vi "Check Channel.vi"(7 "Peripheral":T7, 8 "Error In":errorcluster, 10 "Channels":u8[](array[numeric]), 11 "LINX Resource":T1) -> (0 "Error Out":errorcluster, 2 "Channels":u8[](array[numeric]), 3 "LINX Resource":T1)   [LabVIEW 2014, in "LMH-LINX.lvlib"]
doc: "Generate an error if the specified peripheral channel does not exist on the LINX device."
uses:
  <vilib>/MakerHub/LINX/LMH-LINX.lvlib
  <vilib>/MakerHub/LINX/Private/Type Defs/Peripheral.ctl
  <vilib>/MakerHub/LINX/Private/Type Defs/LINX Ref.ctl
  <vilib>/MakerHub/LINX/Private/Type Defs/Platform.ctl
  <vilib>/MakerHub/LINX/Private/Type Defs/Interface.ctl
  <vilib>/MakerHub/LINX/Private/Device/Type Defs/LINX Device Config.ctl
  <vilib>/MakerHub/LINX/Private/Device/Type Defs/TCP Config.ctl
  <vilib>/MakerHub/LINX/Private/Device/Type Defs/Channels.ctl
  <vilib>/MakerHub/LINX/Private/Type Defs/Error Type.ctl
  <vilib>/MakerHub/LINX/Private/Device/Device.lvlib
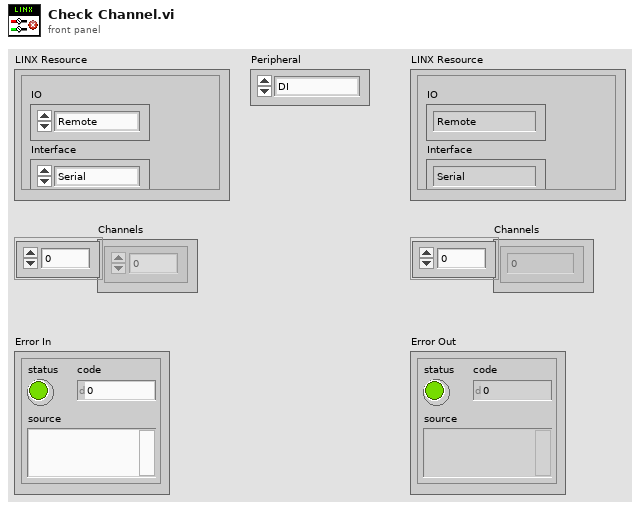
[diagram p1: front panel]
types:
  T1 = typedef "LMH-LINX.lvlib/LINX Ref.ctl" = cluster{"IO":T2, "Interface":T3, "LINX Device Config":T4}
  T2 = typedef "LMH-LINX.lvlib/Platform.ctl" = enum16{"Remote", "Local"}
  T3 = typedef "LMH-LINX.lvlib/Interface.ctl" = enum16{"Serial", "TCP"}
  T4 = typedef "LMH-LINX.lvlib/Device.lvlib/LINX Device Config.ctl" = cluster{"Interface":T3, "COM Port":refnum<visa-resource-name>, "TCP Configuration":T5, "Device Family":u8, "Device ID":u8, "Device Name":string, "TCP Ref":refnum<k5>, "Channels":T6}
  T5 = typedef "LMH-LINX.lvlib/Device.lvlib/TCP Config.ctl" = cluster{"IP Address":string, "Port":u16}
  T6 = typedef "LMH-LINX.lvlib/Channels.ctl" = cluster{"DI":u8[], "DO":u8[], "AI":u8[], "AO":u8[], "PWM":u8[], "QE":u8[], "UART":u8[], "I2C 2":u8[], "SPI":u8[], "CAN":u8[], "Servo":u8[], "AI Ref (V)":dbl, "AI Resolution (Bits)":u8, "AO Ref (V)":dbl, "AO Resolution (Bits)":u8}
  T7 = typedef "LMH-LINX.lvlib/Peripheral.ctl" = enum8{"DI", "DO", "AI", "AO", "PWM", "QE", "UART", "I2C", "SPI", "CAN", "Servo"}
  T8 = typedef "LMH-LINX.lvlib/Error Type.ctl" = enum16{"Unknown", "Timeout", "Corrupt Return Packet", "Unable To Connect", "Command Not Supported", "Channel DNE", "Invalid COM Config", "Firmware Version Mismatch", "myRIO Support", "CMD Specific Error", "Local IO Not Supported"}
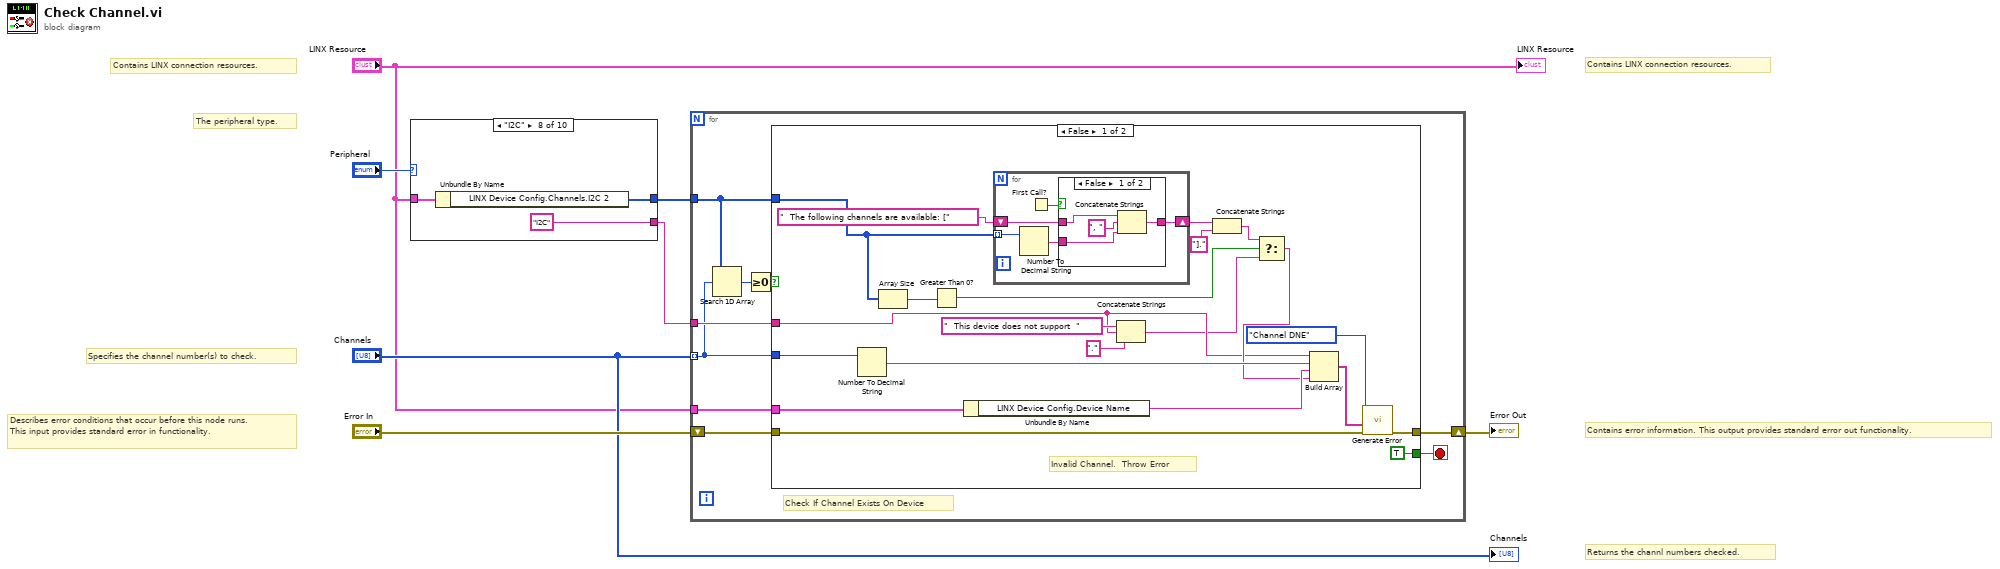
[diagram p0: block diagram]
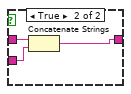
[diagram p2: hidden frame]
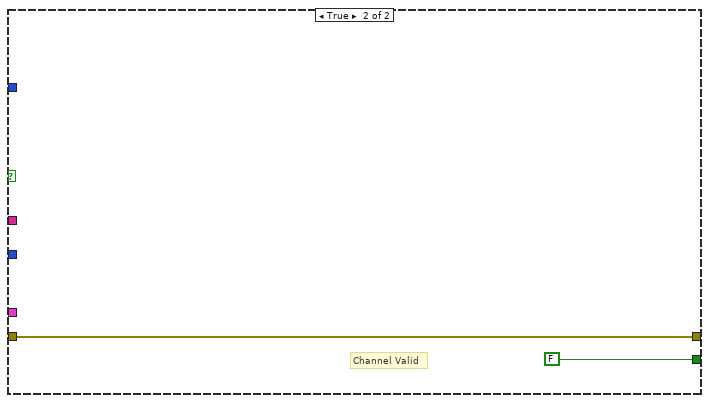
[diagram p3: hidden frame]
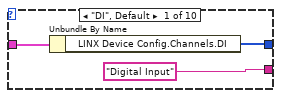
[diagram p4: hidden frame]
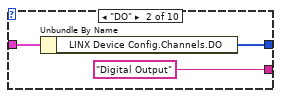
[diagram p5: hidden frame]
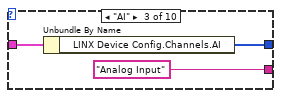
[diagram p6: hidden frame]
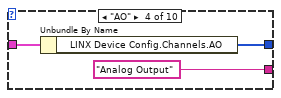
[diagram p7: hidden frame]
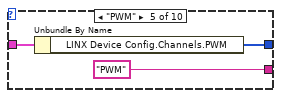
[diagram p8: hidden frame]
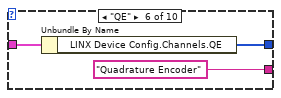
[diagram p9: hidden frame]
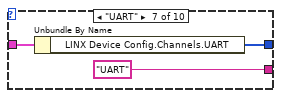
[diagram p10: hidden frame]
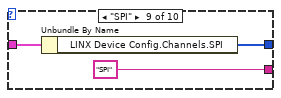
[diagram p11: hidden frame]
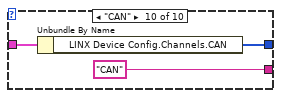
[diagram p12: hidden frame]
diagram:
  # "Returns the channl numbers checked."
  # "Contains LINX connection resources."
  # "Specifies the channel number(s) to check."
  # "The peripheral type."
  # "Contains error information. This output provides standard error out functionality."
  # "Contains LINX connection resources."
  # "Describes error conditions that occur before this node runs. This input provides standard error in functionality."
  n1 = case shown="\"I2C\"" "Peripheral" {
    tunnel: "LINX Resource" -> [w10 w13 w16 w19 w22 w25 w28 w31 w34 w37]
    tunnel: [w9 w12 w15 w18 w21 w24 w27 w30 w33 w36] -> w6
    tunnel: ["Digital Input" "Digital Output" "Analog Input" "Analog Output" "PWM" "Quadrature Encoder" "UART" "I2C" "SPI" "CAN"] -> w4
    frame "DI", Default {
      n2 = Unbundle By Name(w10) -> ("LINX Device Config.Channels.DI"=w9:u8[])
    }
    frame "DO" {
      n3 = Unbundle By Name(w13) -> ("LINX Device Config.Channels.DO"=w12:u8[])
    }
    frame "AI" {
      n4 = Unbundle By Name(w16) -> ("LINX Device Config.Channels.AI"=w15:u8[])
    }
    frame "AO" {
      n5 = Unbundle By Name(w19) -> ("LINX Device Config.Channels.AO"=w18:u8[])
    }
    frame "PWM" {
      n6 = Unbundle By Name(w22) -> ("LINX Device Config.Channels.PWM"=w21:u8[])
    }
    frame "QE" {
      n7 = Unbundle By Name(w25) -> ("LINX Device Config.Channels.QE"=w24:u8[])
    }
    frame "UART" {
      n8 = Unbundle By Name(w28) -> ("LINX Device Config.Channels.UART"=w27:u8[])
    }
    frame "I2C" {
      n9 = Unbundle By Name(w31) -> ("LINX Device Config.Channels.I2C 2"=w30:u8[])
    }
    frame "SPI" {
      n10 = Unbundle By Name(w34) -> ("LINX Device Config.Channels.SPI"=w33:u8[])
    }
    frame "CAN" {
      n11 = Unbundle By Name(w37) -> ("LINX Device Config.Channels.CAN"=w36:u8[])
    }
  }
  n12 = for {
    shift-right: [w44] -> w3
    shift-left: "Error In" -> [w43]
    tunnel: "Channels" -> [w40] mode=indexing
    tunnel: w6 -> [w38]
    tunnel: w4 -> [w41]
    tunnel: "LINX Resource" -> [w39]
    stop <- w42 stop-if-true
    # "Check If Channel Exists On Device"
    n13 = Search 1D Array(1D array=w38, element=w40) -> (index of element=w46:i32)  [unwired: 1 in]
    n14 = Greater Or Equal To 0?(x=w46) -> (x >= 0?=w45:bool)
    n15 = case shown="False" w45 {
      tunnel: [w65 w81] -> w44
      tunnel: w43 -> [w66 w81]
      tunnel: [TRUE FALSE] -> w42
      tunnel: w41 -> [w49 _]
      tunnel: w40 -> [w64 _]
      tunnel: w39 -> [w61 _]
      tunnel: w38 -> [w54 _]
      frame False {
        # "Invalid Channel.  Throw Error"
        n16 = Number To Decimal String(number=w64) -> (decimal integer string=w63:string)  [unwired: 1 in]
        n17 = Array Size(array=w54) -> (size(s)=w53:i32)
        n18 = Greater Than 0?(x=w53) -> (x > 0?=w52:bool)
        n19 = Unbundle By Name(w61) -> ("LINX Device Config.Device Name"=w62:string)
        n20 = for {
          tunnel: w54 -> [w72] mode=indexing
          shift-right: [w68] -> w57
          shift-left: "  The following channels are available: [" ("string") -> [w69]
          n21 = Number To Decimal String(number=w72) -> (decimal integer string=w71:string)  [unwired: 1 in]
          n22 = First Call?() -> (First Call?: T/F=w70:bool)
          n23 = case shown="False" w70 {
            tunnel: w71 -> [w74 w79]
            tunnel: w69 -> [w73 w78]
            tunnel: [w76 w77] -> w68
            frame False {
              n24 = Concatenate Strings(w73, ", " ("string"), w74) -> (w76:string)
            }
            frame True {
              n25 = Concatenate Strings(w78, w79) -> (w77:string)
            }
          }
        }
        n26 = Concatenate Strings("  This device does not support  " ("f"), w49, "." ("string")) -> (w48:string)
        n27 = Concatenate Strings(w57, "]." ("string")) -> (w55:string)
        n28 = Select(t=w55, s=w52, f=w48) -> (s? t:f=w51:string)
        n29 = Build Array(w49, w63, w62, w51) -> (w59:string[])
        n30 = call <vilib>:"Generate Error.vi"("Error In"=w66, "Arguments"=w59, "Error Type"=Error_Type."Channel DNE") -> ("Error Out"=w65:errorcluster)  [unwired: 7 in, 1 out]
      }
      frame True {
        # "Channel Valid"
      }
    }
  }
  "Error Out" <- w3
  "Channels" <- "Channels"
  "LINX Resource" <- "LINX Resource"
